vi "analysis.vi"(6 "Collor":T1, 8 "CS 2":T2(ring), 9 "Direction":enum16{"Zero", "Right", "Front", "Left"}(ring)) -> ()   [LabVIEW 2016]
uses:
  <vilib>/NXT/Subs/LVHSConnector.ctl
  <vilib>/NXT/LegoClasses/BrickReference/BrickReference.lvclass
  <vilib>/NXT/Subs/ColorSensorColors.ctl
  <vilib>/NXT/Dual Mode Library/Display/clearDisplay.vi
  <vilib>/NXT/Dual Mode Library/Display/drawText_Center.vi
panel:
  in  "NXT/EV3":T3
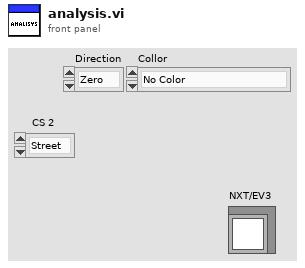
[diagram p1: front panel]
types:
  T1 = typedef "ColorSensorColors.ctl" = enum16{"No Color", "Black", "Blue", "Green", "Yellow", "Red", "White", "Brown"}
  T2 = enum16{"Street", "Intersection", "End", "Stop", "Square", "Delivery"}
  T3 = typedef "LVHSConnector.ctl" = refnum<class "BrickReference.lvclass">
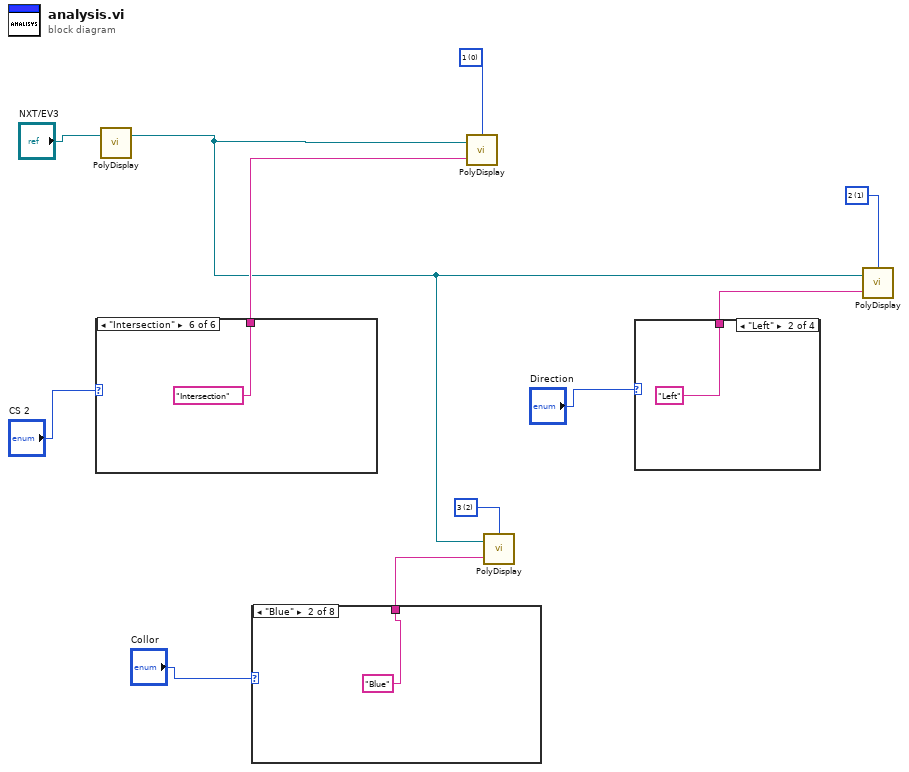
[diagram p0: block diagram]
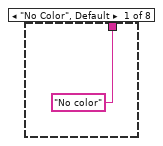
[diagram p2: hidden frame]
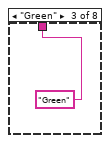
[diagram p3: hidden frame]
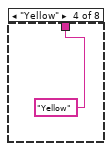
[diagram p4: hidden frame]
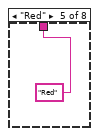
[diagram p5: hidden frame]
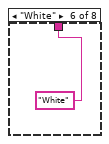
[diagram p6: hidden frame]
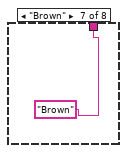
[diagram p7: hidden frame]
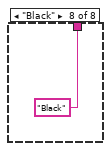
[diagram p8: hidden frame]
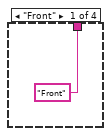
[diagram p9: hidden frame]
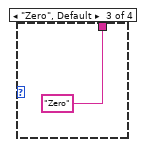
[diagram p10: hidden frame]
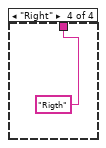
[diagram p11: hidden frame]
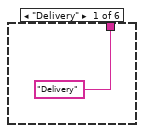
[diagram p12: hidden frame]
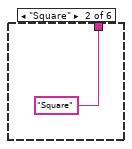
[diagram p13: hidden frame]
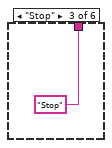
[diagram p14: hidden frame]
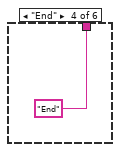
[diagram p15: hidden frame]
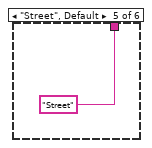
[diagram p16: hidden frame]
diagram:
  w5 = i16 2 items=["1", "2", "3", "4", "5", "6", "7", "8", "9", "10", "11", "12"] ("Line")
  w10 = i16 1 items=["1", "2", "3", "4", "5", "6", "7", "8", "9", "10", "11", "12"] ("Line")
  w11 = i16 0 items=["1", "2", "3", "4", "5", "6", "7", "8", "9", "10", "11", "12"] ("Line")
  n1 = case shown="\"Intersection\"" "CS 2" {
    tunnel: ["Delivery" "Square" "Stop" "End" "Street" "Intersection"] -> w8
    frame "Delivery" {
    }
    frame "Square" {
    }
    frame "Stop" {
    }
    frame "End" {
    }
    frame "Street", Default {
    }
    frame "Intersection" {
    }
  }
  n2 = call-poly <vilib>:"PolyDisplay.vi"("NXT/EV3"="NXT/EV3") -> ("NXT/EV3"=w1:T3)  [unwired: 3 in]
  n3 = case shown="\"Blue\"" "Collor" {
    tunnel: ["No color" "Blue" "Green" "Yellow" "Red" "White" "Brown" "Black"] -> w3
    frame "No Color", Default {
    }
    frame "Blue" {
    }
    frame "Green" {
    }
    frame "Yellow" {
    }
    frame "Red" {
    }
    frame "White" {
    }
    frame "Brown" {
    }
    frame "Black" {
    }
  }
  n4 = call-poly <vilib>:"PolyDisplay.vi"("Text"=w8, "NXT/EV3"=w1, "Line"=w11) -> ()  [unwired: 1 in, 1 out]
  n5 = call-poly <vilib>:"PolyDisplay.vi"("Text"=w3, "NXT/EV3"=w1, "Line"=w5) -> ()  [unwired: 1 in, 1 out]
  n6 = case shown="\"Left\"" "Direction" {
    tunnel: ["Front" "Left" "Zero" "Rigth"] -> w6
    frame "Front" {
    }
    frame "Left" {
    }
    frame "Zero", Default {
    }
    frame "Right" {
    }
  }
  n7 = call-poly <vilib>:"PolyDisplay.vi"("Text"=w6, "NXT/EV3"=w1, "Line"=w10) -> ()  [unwired: 1 in, 1 out]
